vi "FVI_Axes_DeadBand.vi"(10 "deadband Value":dbl, 11 "X axis in":dbl) -> (2 "In Range?":bool, 3 "X axis out":dbl)   [LabVIEW 2018]
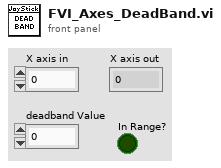
[diagram p1: front panel]
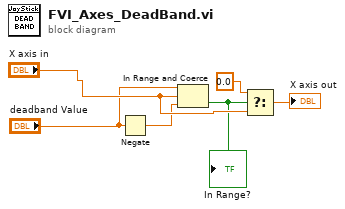
[diagram p0: block diagram]
diagram:
  n1 = Negate(x="deadband Value") -> (-x=w2:dbl)
  n2 = In Range and Coerce(upper limit="deadband Value", x="X axis in", lower limit=w2) -> (In Range?=w3:bool)  [unwired: 1 out]
  "In Range?" <- w3
  n3 = Select(t=0.0 ("x"), s=w3, f="X axis in") -> (s? t:f=→"X axis out":dbl)
